vi "host_for scope.vi"() -> ()   [LabVIEW 2021]
uses:
  <instrlib>/niScope/Acquire/Fetch/niScope Multi Fetch Cluster.vi
  <instrlib>/niScope/Configure/Trigger/niScope Configure Trigger Edge.vi
  <vilib>/Analysis/1siggen.llb/Ramp Pattern by Delta.vi
  <vilib>/Analysis/NI_AALBase.lvlib
panel:
  in  "nex plot":bool
  out "Waveform Graph":T1(graph)
  in  "Channel Name":string="0,1,2,3"
  in  "Resource Name":refnum<k15>="scope" caption="Resource Name(s)"
  in  "pulse amplitude (dB)":dbl=-20.0 format="%#_13g"
  in  "pulse duration (s)":dbl=8e-05 format="%#_13p"
  in  "frequncy comb":cluster{"start":dbl, "end":dbl, "delta":dbl}={"start"=10000000.0, "end"=300000000.0, "delta"=1000000.0} {"delta" format="%#_6p"; "end" format="%#_6p"; "start" format="%#_6p"}
  out "freqency list":dbl[](array[numeric])
  # "Tx state"
  # "Rx state"
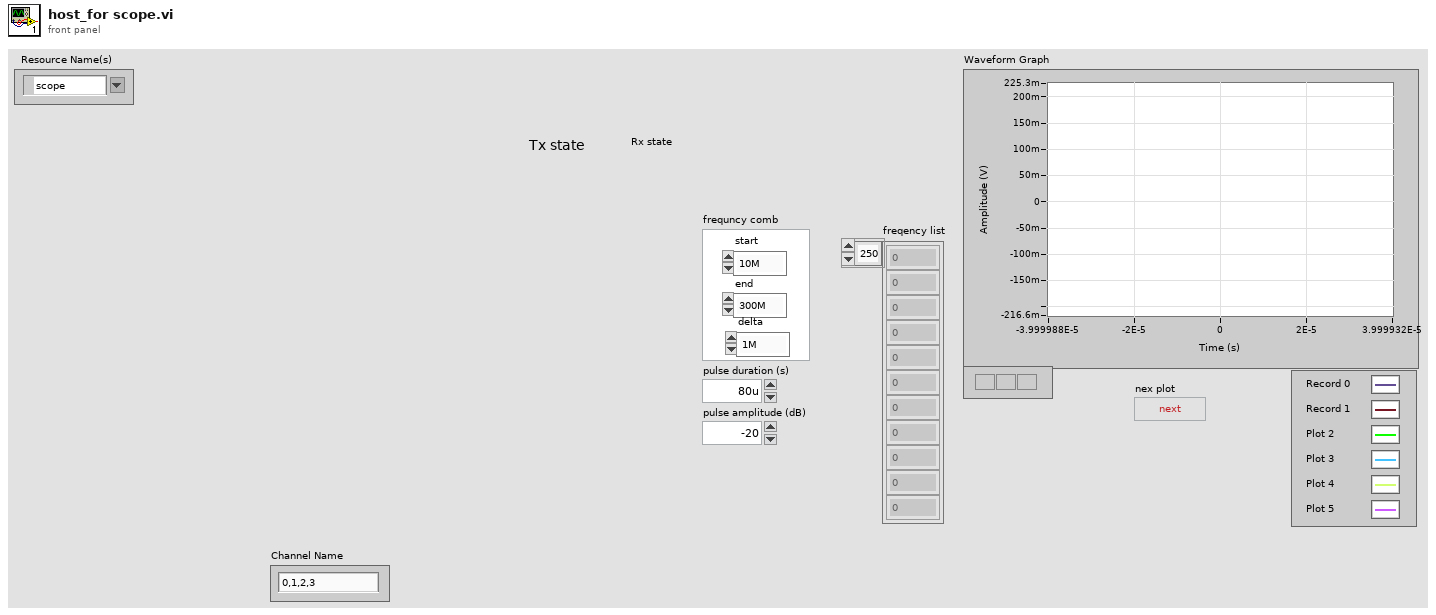
[diagram p1: front panel]
types:
  T1 = cluster{"relativeInitialX":dbl, "xIncrement":dbl, "wfm":dbl[]}[]
  T2 = typedef "PDW_lv2.ctl" = cluster{"t start":dbl, "frequency (Hz)":dbl, "duration (sec)":dbl, "mod type":T3, "mod depth":dbl, "phase (rad)":dbl[], "amp (lin)":dbl[]}
  T3 = typedef "mode_type.ctl" = enum8{"CW", "from memory 1", "NC - cw", "LFM", "BPSK", "QPSK"}
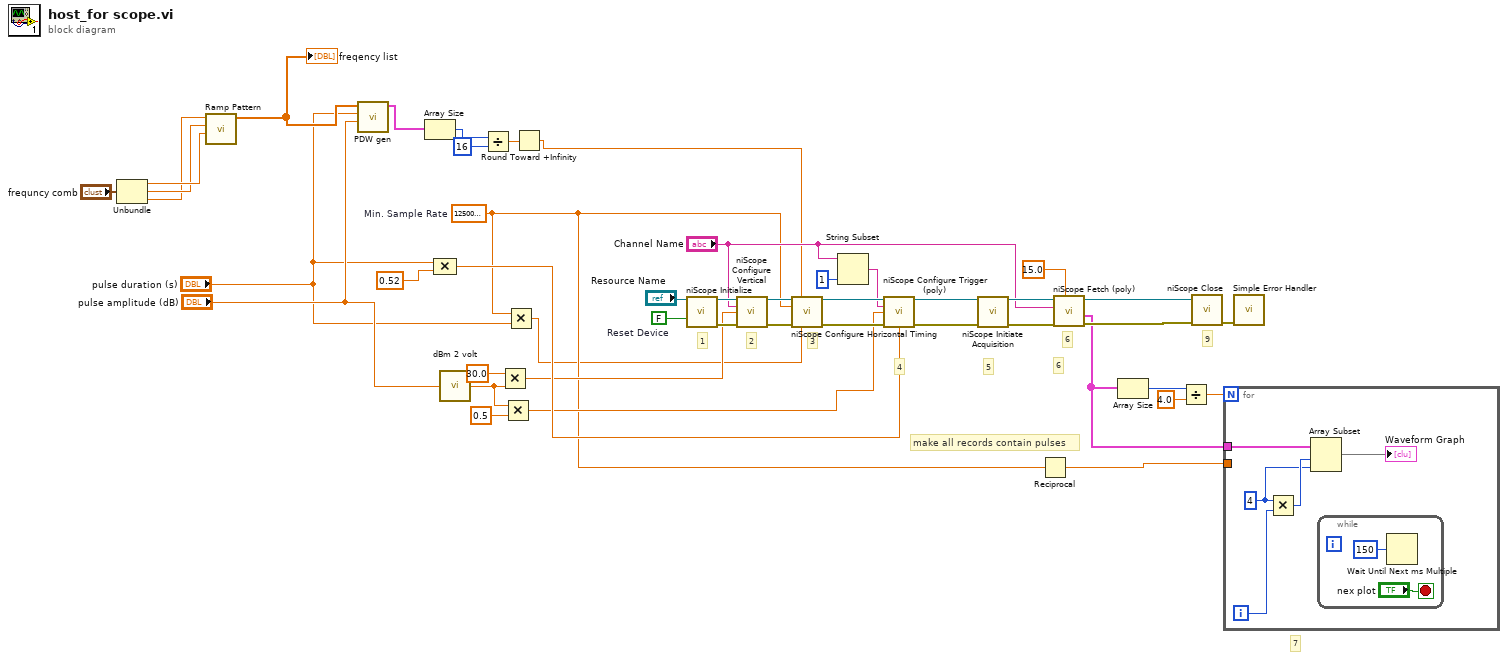
[diagram p0: block diagram]
diagram:
  w4 = 1250000000.0  # Min. Sample Rate
  w40 = FALSE  # Reset Device
  # "make all records contain pulses"
  # "6"
  # "9"
  # "7"
  # "6"
  # "5"
  # "4"
  # "3"
  # "2"
  # "1"
  n1 = Unbundle("frequncy comb") -> ("start"=w44:dbl, "end"=w43:dbl, "delta"=w42:dbl)
  n2 = call-poly <vilib>:"Ramp Pattern.vi"("start"=w44, "end"=w43, "delta"=w42) -> ("Ramp Pattern"=w41:dbl[])  [unwired: 6 in, 2 out]
  "freqency list" <- w41
  n3 = call "PDW gen.vi"("pulse amplitude"="pulse amplitude (dB)", "pulse duration"="pulse duration (s)", "frequency list"=w41) -> ("PDW out"=w26:T2[])  [unwired: 8 in]
  n4 = Array Size(array=w26) -> (size(s)=w25:i32)
  n5 = Compound Arithmetic op=MULTIPLY("pulse duration (s)", 0.52 ("value")) -> (w17:dbl)
  n6 = call "dBm 2 volt.vi"("dBm"="pulse amplitude (dB)") -> ("V"=w8:dbl)
  n7 = Divide(x=w25, y=16) -> (x/y=w23:dbl)
  n8 = Multiply(x=30.0, y=w8) -> (x*y=w5:dbl)
  n9 = Multiply(x=w8, y=0.5) -> (x*y=w6:dbl)
  n10 = Multiply(x=w4, y="pulse duration (s)") -> (x*y=w3:dbl)
  n11 = Round Toward +Infinity(x=w23) -> (ceil(x): smallest int >= x=w1:dbl)
  n12 = call <instrlib>:"niScope Initialize.vi"("resource name"="Resource Name", "reset device"=w40) -> ("instrument handle"=w36:refnum<k15>, "error out"=w35:errorcluster)  [unwired: 12 in]
  n13 = call <instrlib>:"niScope Configure Vertical.vi"("instrument handle"=w36, "channels"="Channel Name", "vertical range"=w5, "error in"=w35) -> ("instrument handle out"=w37:refnum<k15>, "error out"=w38:errorcluster)  [unwired: 10 in]
  n14 = call <instrlib>:"niScope Configure Horizontal Timing.vi"("instrument handle"=w37, "number of records"=w1, "min sample rate"=w4, "error in"=w38, "min record length"=w3) -> ("instrument handle out"=w33:refnum<k15>, "error out"=w34:errorcluster)  [unwired: 9 in]
  n15 = String Subset(string="Channel Name", length (rest)=1 ("length (rest)")) -> (substring=w21:string)  [unwired: 1 in]
  n16 = call-poly <instrlib>:"niScope Configure Trigger (poly).vi"("instrument handle"=w33, "trigger source"=w21, "trigger level"=w6, "error in"=w34, "trigger delay"=w17) -> ("instrument handle out"=w32:refnum<k15>, "error out"=w31:errorcluster)  [unwired: 9 in]
  n17 = call <instrlib>:"niScope Initiate Acquisition.vi"("instrument handle"=w32, "error in"=w31) -> ("instrument handle out"=w30:refnum<k15>, "error out"=w15:errorcluster)  [unwired: 12 in]
  n18 = Reciprocal(x=w4) -> (1/x=w16:dbl)
  n19 = call-poly <instrlib>:"niScope Fetch (poly).vi"("timeout"=15.0, "error in"=w15, "channels"="Channel Name", "instrument handle"=w30) -> ("error out"=w27:errorcluster, "waveform"=w12:T1, "instrument handle out"=w29:refnum<k15>)  [unwired: 4 in, 1 out]
  n20 = Array Size(array=w12) -> (size(s)=w10:i32)
  n21 = Divide(x=w10, y=4.0) -> (x/y=w9:dbl)
  n22 = call <instrlib>:"niScope Close.vi"("instrument handle"=w29, "error in"=w27) -> ("error out"=w28:errorcluster)  [unwired: 13 in]
  n23 = for {
    N: w9 -> [_]
    tunnel: w12 -> [w50]
    tunnel: w16 -> [_]
    i -> [w49]
    w47 = 4 ("x")
    n24 = Multiply(x=w47, y=w49) -> (x*y=w48:i32)
    n25 = Array Subset(array=w50, index=w48, length=w47) -> (→"Waveform Graph":T1)
    n26 = while {
      stop <- "nex plot" stop-if-true
      n27 = Wait Until Next ms Multiple(millisecond multiple=u32 150) -> ()  [unwired: 1 out]
    }
  }
  n28 = call <vilib>:"Simple Error Handler.vi"("error in (no error)"=w28) -> ()  [unwired: 4 in, 5 out]
